vi "Query Audio Devices Example.vi"() -> ()   [LabVIEW 2020]
doc: "An example which demonstrates writing 32-bit floating point data to a WAV file.\n\nSee comments on the block diagram for more information on data types and bit depths."
uses:
  G-Audio.lvlib
panel:
  out "Capture Devices":string[](array[string])
  in  "Refresh":bool
  out "Playback Devices":string[](array[string])
  in  "Available Backends":u16(ring) items=["WASAPI", "DirectSound", "WinMM"]
  out "error out":errorcluster
  # "Instructions:\n1. Run the VI.\n2. Backends will be populated with available audio backends (WASAPI, DirectSound, PulseAudio, etc).\n3. Select a backend. Playback Devices and Capture Devices will be populated with the devices for that backend.\n4. Press the Refresh Devices button to detect any newly added or removed audio devices."
  # "G"
  # "-Audio"
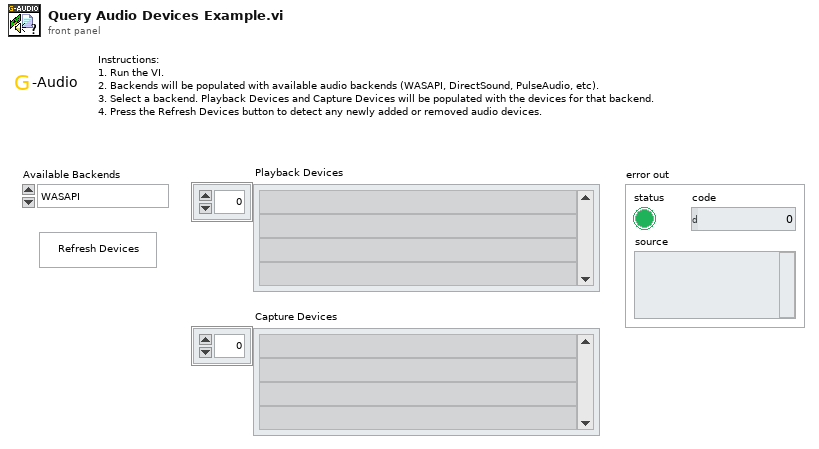
[diagram p1: front panel]
types:
  T1 = typedef "G-Audio.lvlib/Backends.ctl" = enum16{"WASAPI", "DirectSound", "WinMM", "Core Audio", "sndio", "audio(4)", "OSS", "PulseAudio", "ALSA", "JACK", "AAudio", "OpenSL|ES", "Web Audio", "Custom", "Null", "Default"}
  T2 = typedef "G-Audio.lvlib/Audio Device Info.ctl" = cluster{"Name":string, "ID":u8[], "Device Type":T3}
  T3 = typedef "G-Audio.lvlib/Audio Device Type.ctl" = enum16{"(None)", "Playback", "Capture", "Duplex", "Loopback"}
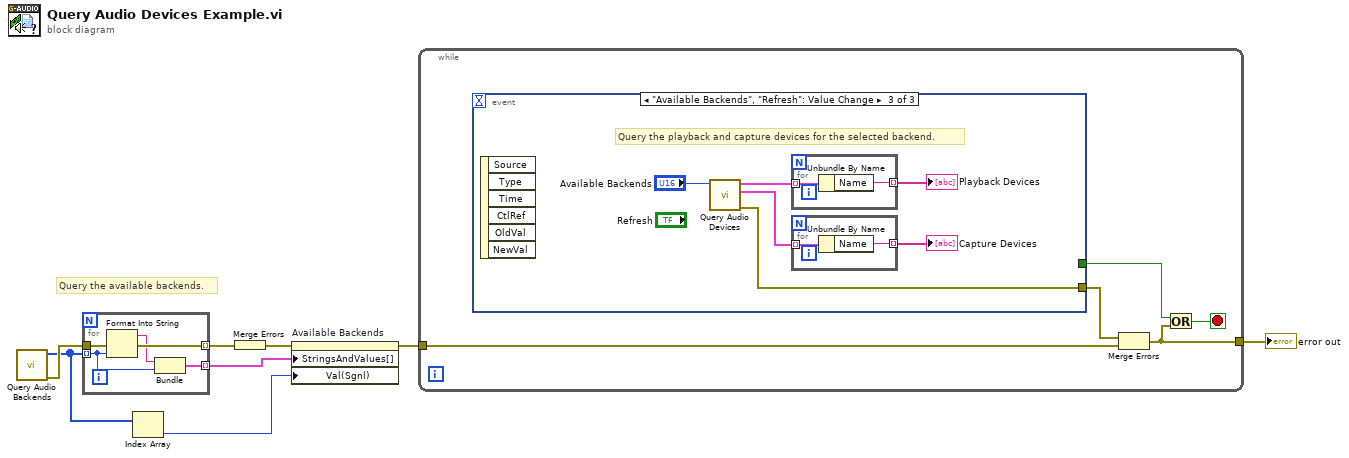
[diagram p0: block diagram]
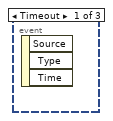
[diagram p2: hidden frame]
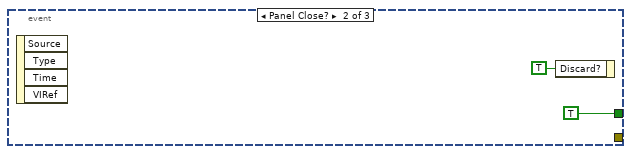
[diagram p3: hidden frame]
diagram:
  # "Query the available backends."
  n1 = call "Query Audio Backends.vi"() -> ("error out"=w7:errorcluster, "Backends"=w3:T1[])  [unwired: 10 in]
  n2 = for {
    tunnel: w3 -> [w10] mode=indexing
    tunnel: w7 -> [w13]
    tunnel: [w12] -> w6 mode=indexing
    tunnel: [w9] -> w4 mode=indexing
    n3 = Format Into String(error in=w13, w10) -> (resulting string=w11:string, error out=w12:errorcluster)  [unwired: 2 in]
    n4 = Bundle(w11, "Backends"=w10) -> (w9:cluster{string, "Backends":T1})  [unwired: 1 in]
  }
  n5 = Index Array(array=w3) -> (element=w2:T1)  [unwired: 1 in]
  n6 = Merge Errors(w6) -> (w5:errorcluster)
  n7 = property on="Available Backends" class="Ring (strict)"(error in=w5, "StringsAndValues[]"=w4, "Val(Sgnl)"=w2) -> (error out=w8:errorcluster)  [unwired: 1 in, 1 out]
  n8 = while {
    tunnel: w8 -> [w18]
    tunnel: [w15] -> w1
    stop <- w16 stop-if-true
    n9 = event shown="[2] \"Available Backends\", \"Refresh\": Value Change" {
      selector: _ -> [_ _ _]
      dyn-events: _ -> [_ _ _]
      timeout: _ -> [_ _ _]
      tunnel: [_ _ w21] -> w17
      tunnel: [_ TRUE _] -> w14
      event Timeout {
        n10 = event-data() -> ()  [unwired: 1 in, 3 out]
      }
      event Panel Close? {
        n11 = event-data() -> ()  [unwired: 1 in, 4 out]
        n12 = event-data("Discard?"=TRUE) -> ()  [unwired: 1 in, 1 out]
      }
      event "Available Backends", "Refresh": Value Change {
        # "Query the playback and capture devices for the selected backend."
        n13 = event-data() -> ()  [unwired: 1 in, 6 out]
        n14 = call "Query Audio Devices.vi"("Backend (Default)"="Available Backends") -> ("error out"=w21:errorcluster, "Capture Devices"=w23:T2[], "Playback Devices"=w25:T2[])  [unwired: 8 in]
        n15 = for {
          tunnel: w25 -> [w30] mode=indexing
          tunnel: [w29] -> w24 mode=indexing
          n16 = Unbundle By Name(w30) -> ("Name"=w29:string)
        }
        "Playback Devices" <- w24
        n17 = for {
          tunnel: w23 -> [w28] mode=indexing
          tunnel: [w27] -> w22 mode=indexing
          n18 = Unbundle By Name(w28) -> ("Name"=w27:string)
        }
        "Capture Devices" <- w22
      }
    }
    n19 = Merge Errors(w17, w18) -> (w15:errorcluster)
    n20 = Or(x=w14, y=w15) -> (x .or. y?=w16:bool)
  }
  "error out" <- w1
